vi "Get_Ref_Launcher.vi"(8 "error in (no error)":errorcluster caption="entrée d'erreur (pas d'erreur)", 11 "Class Popup (Default) en entrée":refnum<class "Class Popup (Main).lvclass">) -> (0 "error out":errorcluster caption="sortie d'erreur", 2 "Ref_Launcher":refnum<vi>, 3 "Class Popup (Default) en sortie":refnum<class "Class Popup (Main).lvclass">)   [LabVIEW 2020, in "Library Instrument & Equipement.lvlib" / "Library Popup.lvlib" / "Class Popup (Main).lvclass"]
uses:
  Class Popup (Main).lvclass
  Class Popup (Main).lvclass/Class Popup (Main).ctl
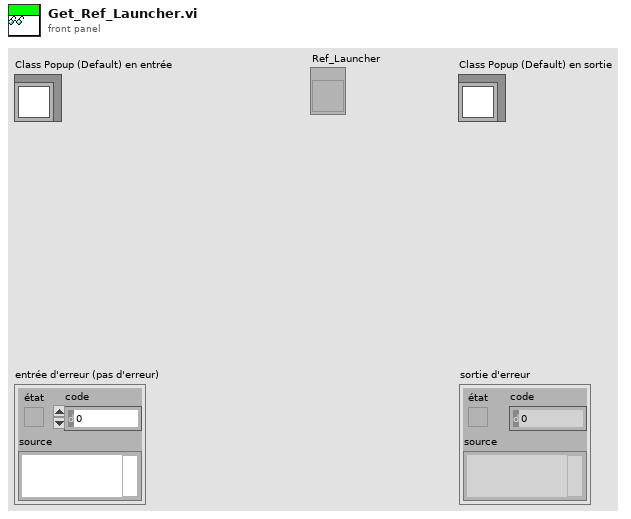
[diagram p1: front panel]
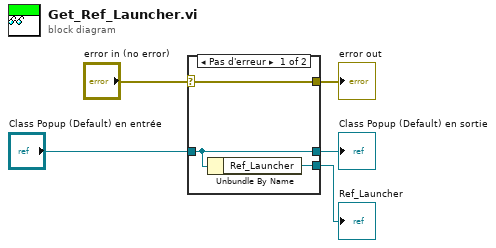
[diagram p0: block diagram]
diagram:
  n1 = case shown="Pas d'erreur" "error in (no error)" {
    selector: "error in (no error)" -> [w8 w9]
    tunnel: [w8 w9] -> w4
    tunnel: [w7 w10] -> w2
    tunnel: "Class Popup (Default) en entrée" -> [w7 w10]
    tunnel: [w6 _] -> w1
    frame No Error {
      n2 = Unbundle By Name(w7) -> ("Ref_Launcher"=w6:refnum<vi>)
    }
    frame Error {
    }
  }
  "error out" <- w4
  "Class Popup (Default) en sortie" <- w2
  "Ref_Launcher" <- w1
